vi "Select_Destination.vi"(8 "error in (no error)":errorcluster, 10 "destTag":string, 11 "IB_DestTree in":refnum<class "IB_Tree_Dest.lvclass">) -> (0 "error out":errorcluster, 3 "IB_DestTree out":refnum<class "IB_Tree_Dest.lvclass">)   [LabVIEW 2020, in "IB_Tree_Dest.lvclass"]
uses:
  <vilib>/AppBuilder/IB_Classes/Tree_Dest/IB_Tree_Dest.lvclass
  <vilib>/AppBuilder/IB_Classes/Tree_Dest/IB_Tree_Dest.lvclass/IB_Tree_Dest.ctl
  <vilib>/AppBuilder/IB_Classes/Tree/IB_Tree.lvclass
  e:/builds/penguin/labview/branches/2020/dev/dist/vi.lib/AppBuilder/IB_Classes/Tree/IB_Tree.lvclass
  e:/builds/penguin/labview/branches/2020/dev/dist/vi.lib/AppBuilder/IB_Classes/Tree_Dest/IB_Tree_Dest.lvclass
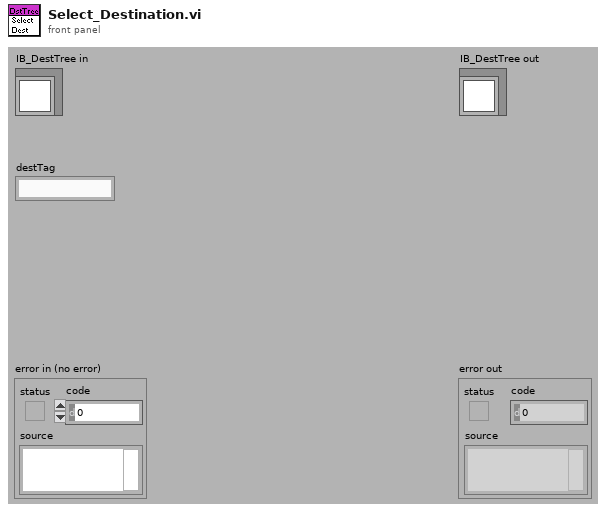
[diagram p1: front panel]
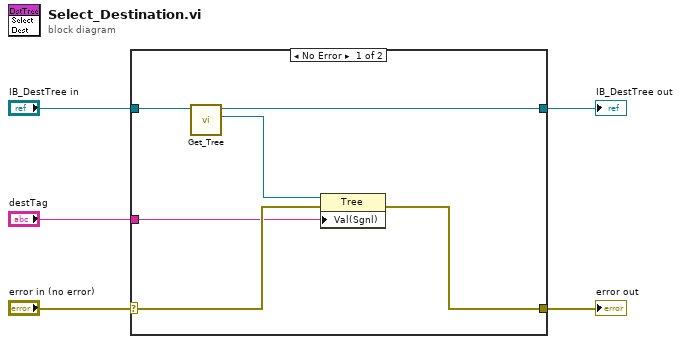
[diagram p0: block diagram]
diagram:
  n1 = case shown="No Error" "error in (no error)" {
    selector: "error in (no error)" -> [w11 w13]
    tunnel: [w10 w13] -> w4
    tunnel: [w8 w12] -> w2
    tunnel: "IB_DestTree in" -> [w9 w12]
    tunnel: "destTag" -> [w6 _]
    frame No Error {
      n2 = call <vilib>:"Get_Tree.vi"("IB_Tree in"=w9) -> ("ctl"=w7:refnum<vi>, "IB_Tree out"=w8:refnum<class "IB_Tree_Dest.lvclass">)  [unwired: 1 in, 8 out]
      n3 = property class="Tree"(reference=w7, error in=w11, "Val(Sgnl)"=w6) -> (error out=w10:errorcluster)  [unwired: 1 out]
    }
    frame Error {
    }
  }
  "error out" <- w4
  "IB_DestTree out" <- w2
